vi "Write String.vi"(8 "error in (no error)":errorcluster, 10 "Value":string, 11 "string in":refnum<class "string.lvclass">) -> (0 "error out":errorcluster, 3 "string out":refnum<class "string.lvclass">)   [LabVIEW 2020, in "Protobuf RAW.lvlib" / "string.lvclass"]
uses:
  string.lvclass
  string.lvclass/string.ctl
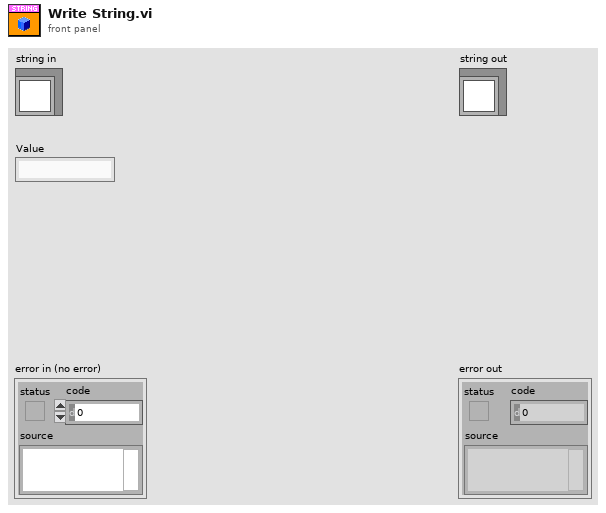
[diagram p1: front panel]
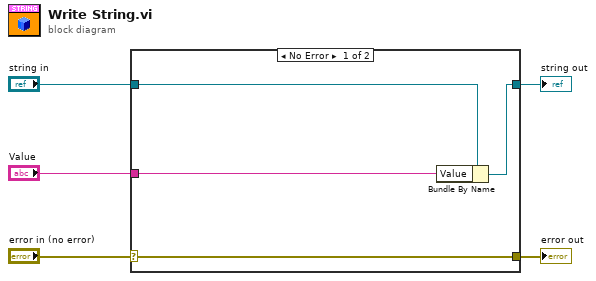
[diagram p0: block diagram]
diagram:
  n1 = case shown="No Error" "error in (no error)" {
    selector: "error in (no error)" -> [w9 w10]
    tunnel: [w9 w10] -> w4
    tunnel: [w7 w11] -> w2
    tunnel: "string in" -> [w8 w11]
    tunnel: "Value" -> [w6 _]
    frame No Error {
      n2 = Bundle By Name(cluster=w8, "Value"=w6) -> (w7:refnum<class "string.lvclass">)
    }
    frame Error {
    }
  }
  "error out" <- w4
  "string out" <- w2
